vi "Control System.vi"(0 "last torque value":dbl, 9 "Sum of error":dbl, 10 "Torque Setpoint":dbl=1.0 format="%#_13g", 11 "Torque  Read":dbl) -> (1 "voltage out":dbl, 2 "Torque Error":dbl)   [LabVIEW 2015]
panel:
  out "accumlated error":dbl
  out "2nd boolean t/f 2":bool
  out "2nd boolean t/f":bool
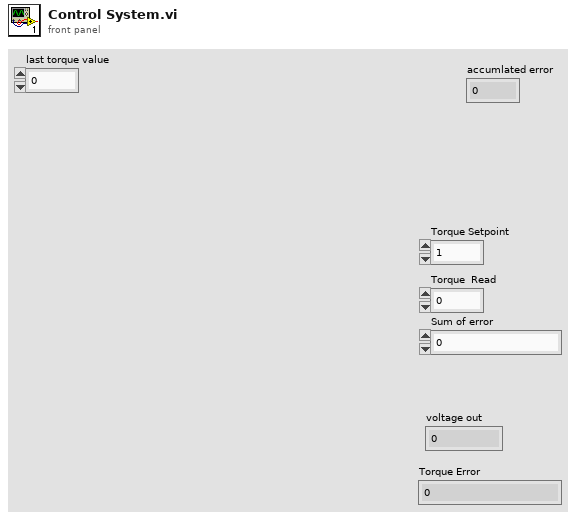
[diagram p1: front panel]
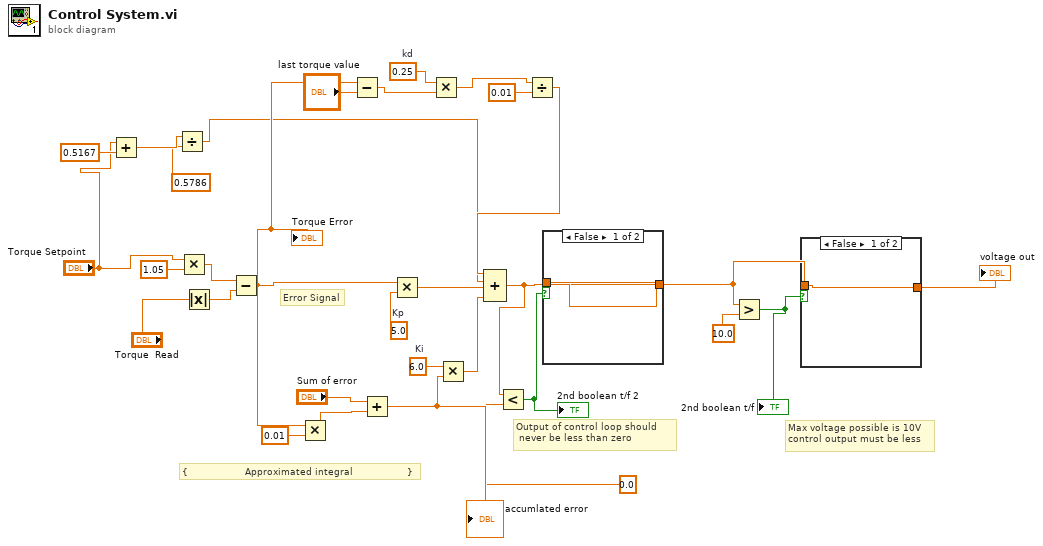
[diagram p0: block diagram]
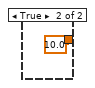
[diagram p2: hidden frame]
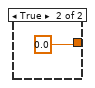
[diagram p3: hidden frame]
diagram:
  w11 = 0.25  # kd
  w26 = 6.0  # Ki
  w31 = 5.0  # Kp
  # "{                   Approximated integral                  }"
  # "Max voltage possible is 10V\ncontrol output must be less"
  # "Output of control loop should\n never be less than zero"
  # "Error Signal"
  n1 = Add(x="Torque Setpoint", y=0.5167) -> (x+y=w5:dbl)
  n2 = Divide(x=w5, y=0.5786) -> (x/y=w6:dbl)
  n3 = Multiply(x="Torque Setpoint", y=1.05) -> (x*y=w1:dbl)
  n4 = Absolute Value(x="Torque  Read") -> (abs(x)=w17:dbl)
  n5 = Subtract(x=w1, y=w17) -> (x-y=w15:dbl)
  "Torque Error" <- w15
  n6 = Multiply(x=w15, y=0.01) -> (x*y=w22:dbl)
  n7 = Subtract(x=w15, y="last torque value") -> (x-y=w12:dbl)
  n8 = Add(x="Sum of error", y=w22) -> (x+y=w24:dbl)
  "accumlated error" <- w24
  n9 = Multiply(x=w15, y=w31) -> (x*y=w25:dbl)
  n10 = Multiply(x=w11, y=w12) -> (x*y=w9:dbl)
  n11 = Multiply(x=w26, y=w24) -> (x*y=w23:dbl)
  n12 = Divide(x=w9, y=0.01) -> (x/y=w8:dbl)
  n13 = Compound Arithmetic op=ADD(w8, w6, w25, w23) -> (w19:dbl)
  n14 = Less?(x=w19, y=0.0) -> (x < y?=w20:bool)
  "2nd boolean t/f 2" <- w20
  n15 = case shown="False" w20 {
    tunnel: [w32 0.0 ("If less than 0.0006")] -> w28
    tunnel: w19 -> [w32 _]
    frame False {
    }
    frame True {
    }
  }
  n16 = Greater?(x=w28, y=10.0) -> (0:w29:bool)
  "2nd boolean t/f" <- w29
  n17 = case shown="False" w29 {
    tunnel: [w34 10.0 ("If less than 0.0006")] -> w27
    tunnel: w28 -> [w34 _]
    frame False {
    }
    frame True {
    }
  }
  "voltage out" <- w27
